vi "3_1.vi"() -> ()   [LabVIEW 2025, in "2022.lvlib"]
uses:
  2022.lvlib
panel:
  out "sum":i32
  out "Array 2":i32[](array[numeric])
  out "Array":string[](array[string])
  out "first subarray":string[](array[string])
  out "second subarray":string[](array[string])
  out "x+1":i32
  out "subarray":string[](array[string])
  out "array 2":string[][](array[string])
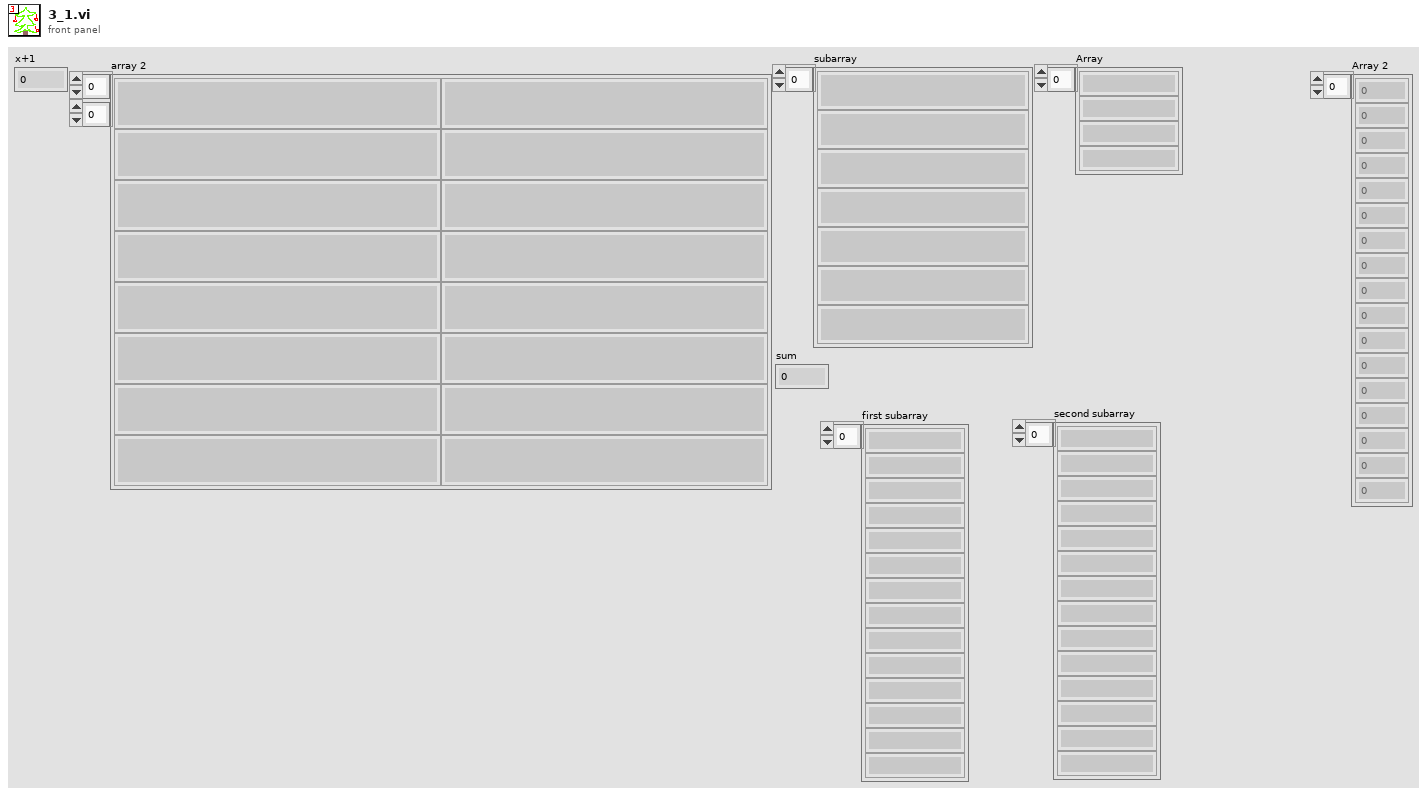
[diagram p1: front panel]
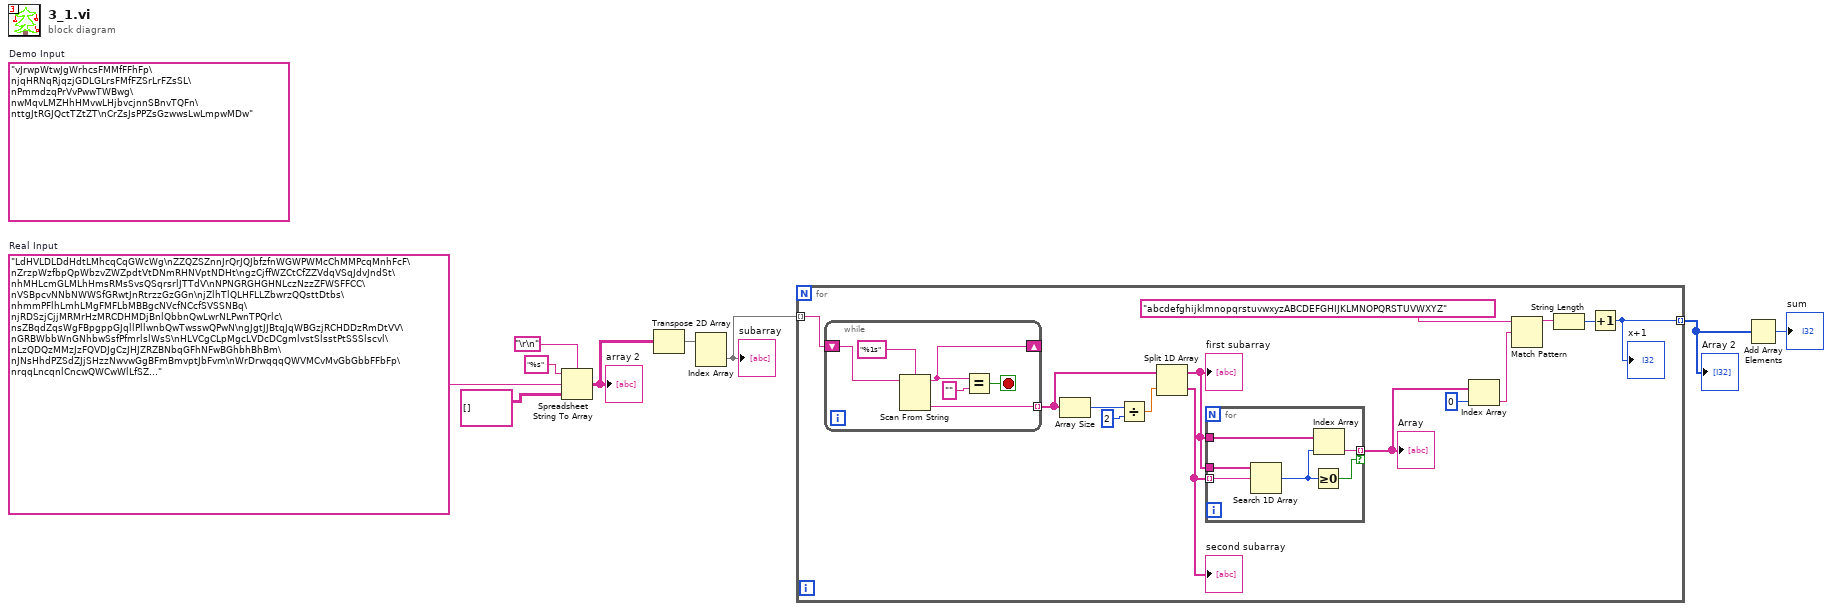
[diagram p0: block diagram]
diagram:
  w1 = "LdHVLDLDdHdtLMhcqCqGWcWg\nZZQZSZnnJrQrJQJbfzfnWGWPWMcChMMPcqMnhFcF\nZrzpWzfbpQpWbzvZWZpdtVtDNmRHNVptNDHt\ngzCjffWZCtCfZZVdqVSqJdvJndSt\nhMHLcmGLMLhHmsRMsSvsQSqrsrlJTTdV\nNPNGRGHGHNLczNzzZFWSFFCC\nVSBpcvNNbNWWSfGRwtJnRtrzzGzGGn\njZlhTlQLHFLLZbwrzQQsttDtbs\nhmmPFlhLmhLMgFMFLbMBBgcNVcfNCcfSVSSNBq\njRDSzjCjjMRMrHzMRCDHMDjBnlQbbnQwLwrNLPwnTPQrlc\nsZBqdZqsWgFBpgppGJqllPllwnbQwTwsswQPwN\ngJgtJJBtqJqWBGzjRCHDDzRmDtVV\nGRBWbbWnGNhbwSsfPfmrlslWsS\nHLVCgCLpMgcLVDcDCgmlvstSlsstPtSSSlscvl\nLzQDQzMMzJzFQVDJgCzJHJZRZBNbqGFhNFwBGhbhBhBm\nJNsHhdPZSdZJjSHzzNwvwGgBFmBmvptJbFvm\nWrDrwqqqQWVMCvMvGbGbbFFbFp\nrqqLncqnlCncwQWCwWlLfSZ..."  # Real Input
  (unwired) "vJrwpWtwJgWrhcsFMMfFFhFp\njqHRNqRjqzjGDLGLrsFMfFZSrLrFZsSL\nPmmdzqPrVvPwwTWBwg\nwMqvLMZHhHMvwLHjbvcjnnSBnvTQFn\nttgJtRGJQctTZtZT\nCrZsJsPPZsGzwwsLwLmpwMDw"  # Demo Input
  n1 = Spreadsheet String To Array(delimiter (Tab)="\r\n", format string="%s", spreadsheet string=w1, array type (2D Dbl)=string[][] []) -> (array=w6:string[][])
  "array 2" <- w6
  n2 = Transpose 2D Array(2D array=w6) -> (transposed array=w5:string[][])
  n3 = Index Array(array=w5) -> (element=w4:string[])  [unwired: 2 in]
  "subarray" <- w4
  n4 = for {
    tunnel: w4 -> [w23] mode=indexing
    tunnel: [w12] -> w3 mode=indexing
    n5 = while {
      shift-right: [w32] -> _
      shift-left: w23 -> [w35]
      tunnel: [w30] -> w20 mode=indexing
      stop <- w33 stop-if-true
      n6 = Scan From String(format string="%1s", input string=w35) -> (remaining string=w32:string, output 1=w30:string)  [unwired: 3 in, 2 out]
      n7 = Equal?(x=w32, y="") -> (x = y?=w33:bool)
    }
    n8 = Array Size(array=w20) -> (size(s)=w22:i32)
    n9 = Divide(x=w22, y=2) -> (x/y=w19:dbl)
    n10 = Split 1D Array(array=w20, index=w19) -> (first subarray=w18:string[], second subarray=w17:string[])
    "second subarray" <- w17
    "first subarray" <- w18
    n11 = for {
      tunnel: w17 -> [w29] mode=indexing
      tunnel: w18 -> [w26]
      tunnel: w18 -> [w28]
      tunnel: [w24] -> w10 mode=indexing if=w27
      n12 = Search 1D Array(1D array=w28, element=w29) -> (index of element=w25:i32)  [unwired: 1 in]
      n13 = Greater Or Equal To 0?(x=w25) -> (x >= 0?=w27:bool)
      n14 = Index Array(array=w26, index=w25) -> (element=w24:string)
    }
    "Array" <- w10
    n15 = Index Array(array=w10, index=0) -> (element=w11:string)
    n16 = Match Pattern(string="abcdefghijklmnopqrstuvwxyzABCDEFGHIJKLMNOPQRSTUVWXYZ" ("y"), regular expression=w11) -> (before substring=w15:string)  [unwired: 1 in, 3 out]
    n17 = String Length(string=w15) -> (length=w16:i32)
    n18 = Increment(x=w16) -> (x+1=w12:i32)
    "x+1" <- w12
  }
  "Array 2" <- w3
  n19 = Add Array Elements(numeric array=w3) -> (sum=→"sum":i32)
